vi "Param Decode.vi"(7 "index":i32=6, 8 "error in (no error)":errorcluster, 10 "Array - letter":string[](array[string])) -> (0 "error out":errorcluster, 2 "Array -parameter":string[](array[string]))   [LabVIEW 2021, in "STAV lib.lvlib"]
uses:
  STAV lib.lvlib
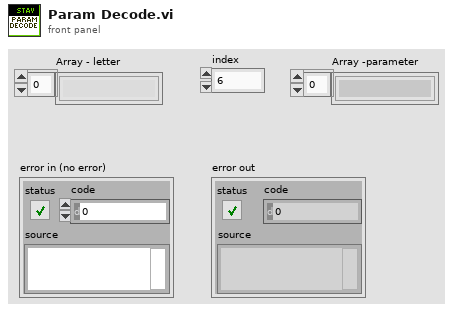
[diagram p1: front panel]
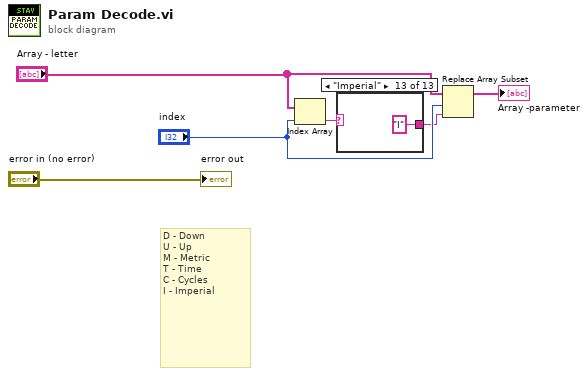
[diagram p0: block diagram]
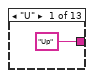
[diagram p2: hidden frame]
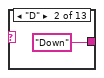
[diagram p3: hidden frame]
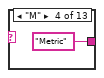
[diagram p5: hidden frame]
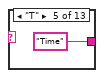
[diagram p6: hidden frame]
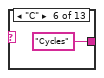
[diagram p7: hidden frame]
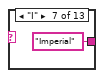
[diagram p8: hidden frame]
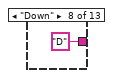
[diagram p9: hidden frame]
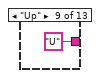
[diagram p10: hidden frame]
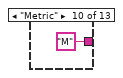
[diagram p11: hidden frame]
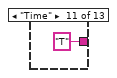
[diagram p12: hidden frame]
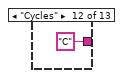
[diagram p13: hidden frame]
diagram:
  # "D - Down\nU - Up\nM - Metric\nT - Time\nC - Cycles\nI - Imperial"
  n1 = Index Array(array="Array - letter", index="index") -> (element=w6:string)
  n2 = case shown="\"Imperial\"" w6 {
    selector: w6 -> [_ _ w9 _ _ _ _ _ _ _ _ _ _]
    tunnel: ["Up" "Down" w9 "Metric" "Time" "Cycles" "Imperial" "D" "U" "M" "T" "C" "I"] -> w4
    frame "U" {
    }
    frame "D" {
    }
    frame "none", Default {
    }
    frame "M" {
    }
    frame "T" {
    }
    frame "C" {
    }
    frame "I" {
    }
    frame "Down" {
    }
    frame "Up" {
    }
    frame "Metric" {
    }
    frame "Time" {
    }
    frame "Cycles" {
    }
    frame "Imperial" {
    }
  }
  n3 = Replace Array Subset(array="Array - letter", new element=w4, index="index") -> (→"Array -parameter":string[])
  "error out" <- "error in (no error)"
